vi "Open File.vi"(8 "error in (no error)":errorcluster, 11 "Spectrum Recorder in":refnum<class "Spectrum Recorder too.lvclass">) -> (0 "error out":errorcluster, 3 "Spectrum Recorder out":refnum<class "Spectrum Recorder too.lvclass">)   [LabVIEW 2024, in "Spectrum Recorder too.lvclass"]
uses:
  Spectrum Recorder too.lvclass
  Spectrum Recorder too.lvclass/Spectrum Recorder too.ctl
  Controllers/Application Controller Messages/New Data File Msg/New Data File Msg.lvclass
  <vilib>/ActorFramework/Actor/Actor.lvclass
  Plots/Plot types.ctl
  NHMFL_Core/Libraries/Red Pitaya/RP Core/Red Pitaya Transceiver Driver/Internal Spectrum Configuration.ctl
  Loggers/Logger/Logger.lvclass
  C:/Git/LabActor/Recorders/Continuous Recorder Actor/Continuous Recorder Actor.lvclass
  C:/Git/LabActor/Instrument Actor/Instrument Actor.lvclass
  C:/Git/LabActor/Worker/Worker Actor/Worker Actor.lvclass
  C:/Git/LabActor/Template Module/Template Module.lvclass
  C:/Program Files/National Instruments/LabVIEW 2024/vi.lib/ActorFramework/Actor/Actor.lvclass
  C:/Git/LabActor/Worker/Woker Interface/Worker.lvclass
  C:/Git/LabActor/Recorders/Interfaces/Continuous Recorder/Continuous Recorder.lvclass
  C:/Git/LabActor/Spectrum Recorder too/Spectrum Recorder too.lvclass
  C:/Git/LabActor/Publish-Subscribe/Interfaces/Subscriber/Subscriber.lvclass
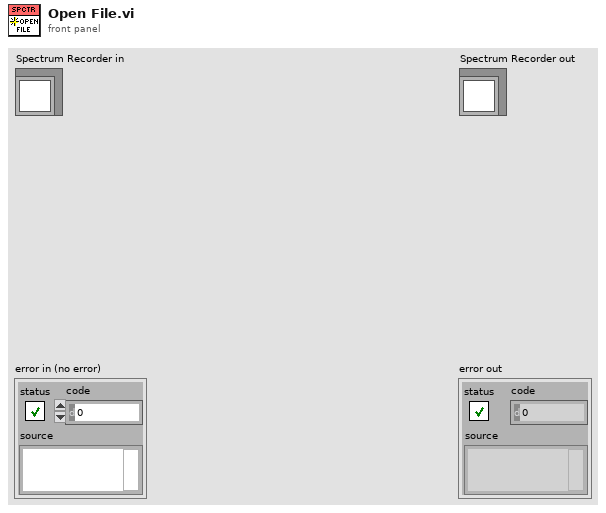
[diagram p1: front panel]
types:
  T1 = typedef "Plot types.ctl" = enum16{"Waveform Plot", "XY Plot", "Full XY"}
  T2 = typedef "Internal Spectrum Configuration.ctl" = cluster{"Start frequency":dbl, "End frequency":dbl, "Coarse step":dbl, "Step duration":dbl, "Red Pitaya address":string, "Open plot \non start":bool, "Fine region centers":dbl[], "Regions width":dbl, "Fine step":dbl, "Pause between scans":dbl, "Clear rgs on start":bool, "Output amplitude":dbl}
  T3 = typedef "Spectrum Configuration.ctl" = cluster{"Start frequency":dbl, "End frequency":dbl, "Coarse step":dbl, "Step duration":dbl, "Red Pitaya address":string, "Open plot \non start":bool, "Regions width":dbl, "Fine step":dbl, "Pause between scans":dbl, "Clear rgs on start":bool, "Output amplitude":dbl, "Append measurements":string[], "Full scan period":dbl, "Full start":dbl, "Full end":dbl, "Full step":dbl}
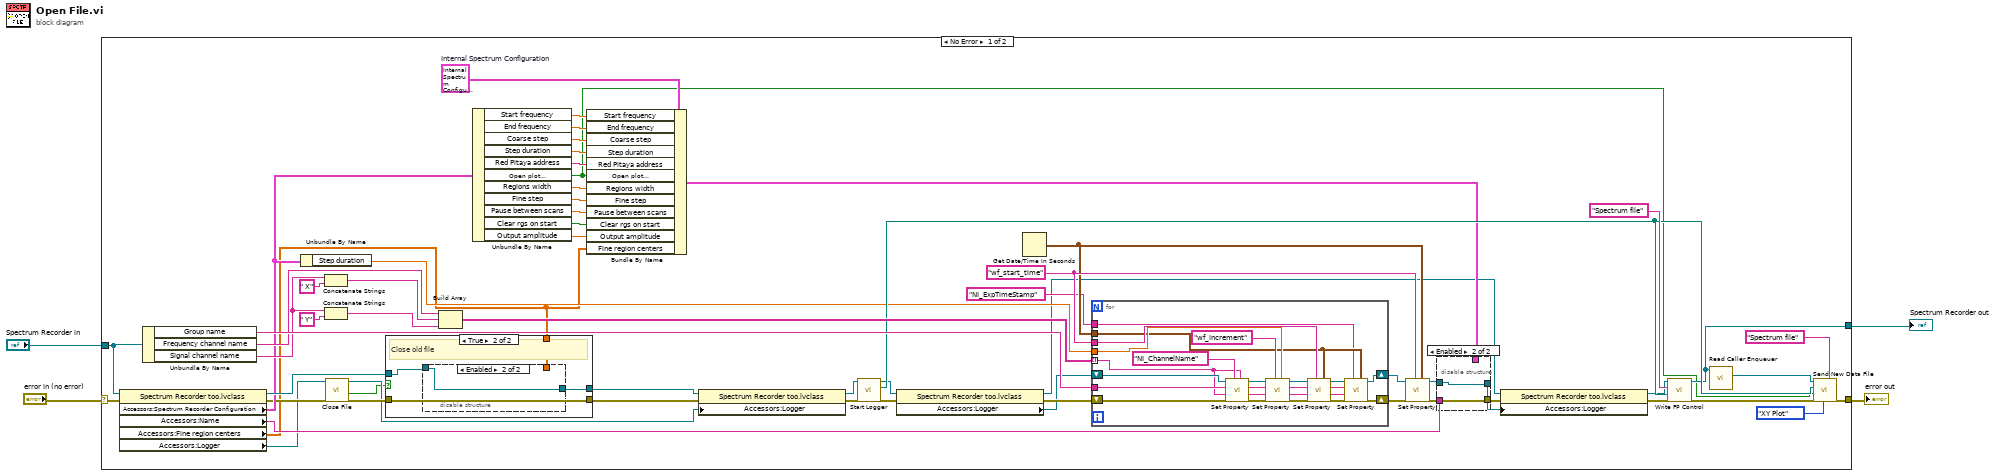
[diagram p0: block diagram]
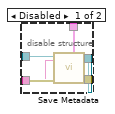
[diagram p2: hidden frame]
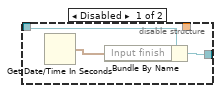
[diagram p4: hidden frame]
diagram:
  n1 = case shown="No Error" "error in (no error)" {
    selector: "error in (no error)" -> [w63 w109]
    tunnel: [w49 w109] -> w3
    tunnel: [w46 w108] -> w1
    tunnel: "Spectrum Recorder in" -> [w62 w108]
    frame No Error {
      w35 = T2 {"Start frequency"=500000.0, "End frequency"=2000000.0, "Coarse step"=100.0, "Step duration"=0.004, "Red Pitaya address"="192.168.1.100", "Open plot \non start"=FALSE, "Fine region centers"=[], "Regions width"=2000.0, "Fine step"=1.0, "Pause between scans"=0.0, "Clear rgs on start"=FALSE, "Output amplitude"=1.0}  # Internal Spectrum Configuration
      w38 = "wf_start_time"
      n2 = property class="Spectrum Recorder too.lvclass"(reference=w62, error in=w63) -> (reference out=w59:refnum<class "Spectrum Recorder too.lvclass">, error out=w13:errorcluster, "Accessors:Spectrum Recorder Configuration"=w34:T3, "Accessors:Name"=w19:string, "Accessors:Fine region centers"=w5:dbl[], "Accessors:Logger"=w11:refnum<class "Logger.lvclass">)
      n3 = Unbundle By Name(w62) -> ("Group name"=w65:string, "Frequency channel name"=w64:string, "Signal channel name"=w54:string)
      n4 = Unbundle By Name(w34) -> ("Step duration"=w43:dbl)
      n5 = Concatenate Strings(w54, " X" ("string")) -> (w55:string)
      n6 = Concatenate Strings(w54, " Y" ("string")) -> (w53:string)
      n7 = call-dynamic "Close File.vi"("error in (no error)"=w13, "Logger in"=w11) -> ("error out"=w12:errorcluster, "Actually closed"=w6:bool, "Logger out"=w7:refnum<class "Logger.lvclass">)  [unwired: 6 in, 1 out]
      n8 = case shown="True" w6 {
        tunnel: w12 -> [w99 w101]
        tunnel: [w99 w101] -> w60
        tunnel: w59 -> [w98 w103]
        tunnel: [w98 w102] -> w9
        tunnel: w5 -> [_ w100]
        frame False {
        }
        frame True {
          # "Close old file"
          n9 = disable-structure shown="Enabled" {
            disable-tunnel: w103 -> [w106 w107]
            disable-tunnel: [w105 w107] -> w102
            disable-tunnel: w100 -> [_ _]
            frame Disabled {
              n10 = Get Date/Time In Seconds() -> (seconds since 1Jan1904=w104:timestamp)
              n11 = Bundle By Name(cluster=w106, "Input finish"=w104) -> (w105:refnum<class "Spectrum Recorder too.lvclass">)
            }
            frame Enabled {
            }
          }
        }
      }
      n12 = Build Array(w64, w55, w53) -> (w61:string[])
      n13 = Unbundle By Name(w34) -> ("Start frequency"=w33:dbl, "End frequency"=w32:dbl, "Coarse step"=w31:dbl, "Step duration"=w30:dbl, "Red Pitaya address"=w29:string, "Open plot \non start"=w14:bool, "Regions width"=w28:dbl, "Fine step"=w27:dbl, "Pause between scans"=w26:dbl, "Clear rgs on start"=w25:bool, "Output amplitude"=w24:dbl)
      n14 = Bundle By Name(cluster=w35, "Start frequency"=w33, "End frequency"=w32, "Coarse step"=w31, "Step duration"=w30, "Red Pitaya address"=w29, "Open plot \non start"=w14, "Regions width"=w28, "Fine step"=w27, "Pause between scans"=w26, "Clear rgs on start"=w25, "Output amplitude"=w24, "Fine region centers"=w5) -> (w23:T2)
      n15 = property class="Spectrum Recorder too.lvclass"(reference=w9, error in=w60, "Accessors:Logger"=w7) -> (reference out=w8:refnum<class "Spectrum Recorder too.lvclass">, error out=w10:errorcluster)
      n16 = call-dynamic "Start Logger.vi"("error in (no error)"=w10, "Worker in"=w8) -> ("error out"=w58:errorcluster, "File Path"=w48:path, "Worker out"=w21:refnum<class "Spectrum Recorder too.lvclass">)  [unwired: 6 in, 1 out]
      n17 = property class="Spectrum Recorder too.lvclass"(reference=w21, error in=w58) -> (reference out=w17:refnum<class "Spectrum Recorder too.lvclass">, error out=w22:errorcluster, "Accessors:Logger"=w20:refnum<class "Logger.lvclass">)
      n18 = Get Date/Time In Seconds() -> (seconds since 1Jan1904=w37:timestamp)
      n19 = for {
        tunnel: w65 -> [w96]
        tunnel: w61 -> [w93] mode=indexing
        shift-right: [w78] -> w40
        shift-left: w20 -> [w97]
        shift-right: [w79] -> w42
        shift-left: w22 -> [w95]
        tunnel: w43 -> [w83]
        tunnel: w37 -> [w77]
        tunnel: w38 -> [w82]
        tunnel: "NI_ExpTimeStamp" -> [w76]
        n20 = call-dynamic "Set Property.vi"("property value"=w93, "property name"="NI_ChannelName", "error in (no error)"=w95, "channel name"=w93, "group name"=w96, "Logger in"=w97) -> ("error out"=w92:errorcluster, "channel name out"=w87:string, "group name out"=w88:string, "Logger out"=w91:refnum<class "Logger.lvclass">)  [unwired: 2 in]
        n21 = call-dynamic "Set Property.vi"("property value"=w83, "property name"="wf_increment", "error in (no error)"=w92, "channel name"=w87, "group name"=w88, "Logger in"=w91) -> ("error out"=w89:errorcluster, "channel name out"=w86:string, "group name out"=w85:string, "Logger out"=w90:refnum<class "Logger.lvclass">)  [unwired: 2 in]
        n22 = call-dynamic "Set Property.vi"("property value"=w77, "property name"=w82, "error in (no error)"=w89, "channel name"=w86, "group name"=w85, "Logger in"=w90) -> ("error out"=w80:errorcluster, "channel name out"=w74:string, "group name out"=w75:string, "Logger out"=w81:refnum<class "Logger.lvclass">)  [unwired: 2 in]
        n23 = call-dynamic "Set Property.vi"("property value"=w77, "property name"=w76, "error in (no error)"=w80, "channel name"=w74, "group name"=w75, "Logger in"=w81) -> ("error out"=w79:errorcluster, "Logger out"=w78:refnum<class "Logger.lvclass">)  [unwired: 2 in, 2 out]
      }
      n24 = call-dynamic "Set Property.vi"("property value"=w37, "property name"=w38, "error in (no error)"=w42, "Logger in"=w40) -> ("error out"=w41:errorcluster, "Logger out"=w39:refnum<class "Logger.lvclass">)  [unwired: 4 in, 2 out]
      n25 = disable-structure shown="Enabled" {
        disable-tunnel: [w71 w72] -> w52
        disable-tunnel: w41 -> [w70 w72]
        disable-tunnel: w39 -> [w69 w73]
        disable-tunnel: w23 -> [w68 _]
        disable-tunnel: w19 -> [w67 _]
        disable-tunnel: [w66 w73] -> w16
        frame Disabled {
          n26 = call-dynamic "Save Metadata.vi"(5:w68, 7:w67, "error in (no error)"=w70, "Logger in"=w69) -> ("error out"=w71:errorcluster, "Logger out"=w66:refnum<class "Logger.lvclass">)  [unwired: 4 in, 2 out]
        }
        frame Enabled {
        }
      }
      n27 = property class="Spectrum Recorder too.lvclass"(reference=w17, error in=w52, "Accessors:Logger"=w16) -> (reference out=w15:refnum<class "Spectrum Recorder too.lvclass">, error out=w18:errorcluster)
      n28 = call-dynamic "Write FP Control.vi"("error in (no error)"=w18, "Control Value"=w48, "Control Name"="Spectrum file", "Measure Object in"=w15) -> ("error out"=w47:errorcluster, "Measure Object out"=w46:refnum<class "Spectrum Recorder too.lvclass">)  [unwired: 6 in]
      n29 = call <vilib>:"Read Caller Enqueuer.vi"("Actor"=w46) -> ("Caller Enqueuer"=w50:refnum<class "Message Enqueuer.lvclass">)  [unwired: 10 in]
      n30 = call "Send New Data File.vi"("Plot group"="Spectrum file", "Plot type"=Plot_types."XY Plot", "error in (no error)"=w47, "New plot if not open"=w14, "File"=w48, "Message Enqueuer"=w50) -> ("error out"=w49:errorcluster)  [unwired: 4 in, 1 out]
    }
    frame Error {
    }
  }
  "error out" <- w3
  "Spectrum Recorder out" <- w1
